vi "Update Custom Parameters.vi"(6 "Assert VI":path, 8 "error in (no error)":errorcluster, 10 "New Data Type":path) -> (0 "error out":errorcluster)   [LabVIEW 2018]
doc: "Updates the data types in the custom cluster data type, avoids having a whole set of extra type defs to maintain for the GTLT tests"
uses:
  <vilib>/Utility/traverseref.llb/TRef TravTarget.ctl
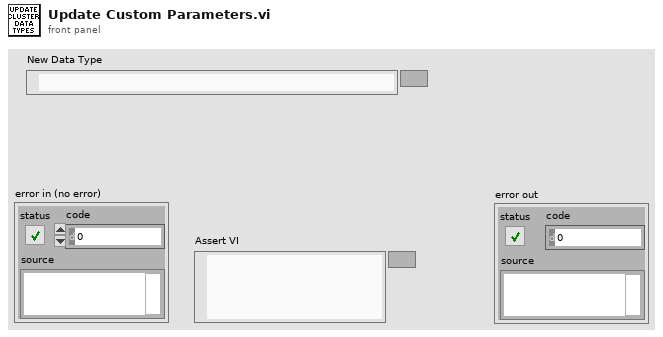
[diagram p1: front panel]
types:
  T1 = typedef "TRef TravTarget.ctl" = enum16{"FP", "BD", "Other"}
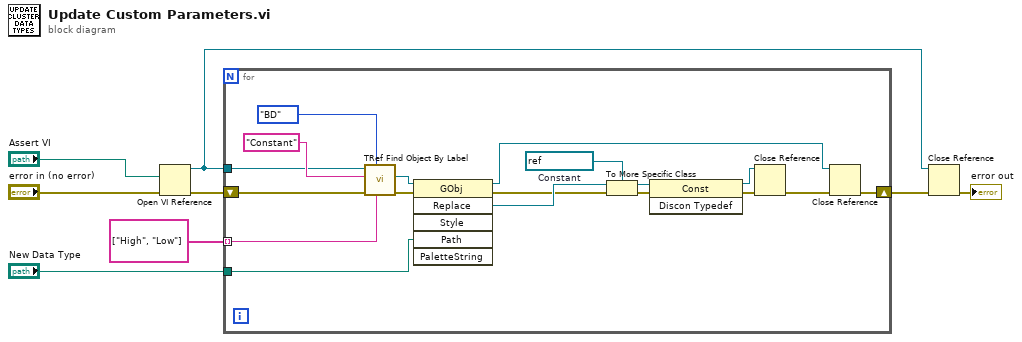
[diagram p0: block diagram]
diagram:
  n1 = Open VI Reference(vi path="Assert VI", error in (no error)="error in (no error)") -> (vi reference=w1:refnum<vi>, error out=w5:errorcluster)  [unwired: 4 in]
  n2 = for {
    tunnel: string[] ["High", "Low"] ("Label") -> [w26] mode=indexing
    tunnel: "New Data Type" -> [w21]
    tunnel: w1 -> [w9]
    shift-right: [w13] -> w3
    shift-left: w5 -> [w14]
    w19 = refnum<vi> refnum  # Constant
    n3 = call <vilib>:"TRef Find Object By Label.vi"("Label"=w26, "Traverse Target"=TRef_TravTarget."BD", "error in (no error)"=w14, "Class Name"="Constant", "VI Ref"=w9) -> ("error out"=w22:errorcluster, "Found Obj Ref"=w23:refnum<vi>)  [unwired: 3 in, 2 out]
    n4 = invoke class="GObj" method="Replace"(reference=w23, error in=w22, "Path"=w21) -> (reference out=w11:refnum<vi>, error out=w16:errorcluster, "Replace"=w20:refnum<vi>)  [unwired: 3 in, 3 out]
    n5 = To More Specific Class(target class=w19, reference=w20, error in=w16) -> (specific class reference=w18:refnum<vi>, error out=w17:errorcluster)
    n6 = invoke class="Const" method="Discon Typedef"(reference=w18, error in=w17) -> (reference out=w10:refnum<vi>, error out=w15:errorcluster)  [unwired: 1 in, 1 out]
    n7 = Close Reference(reference=w10, error in (no error)=w15) -> (error out=w12:errorcluster)
    n8 = Close Reference(reference=w11, error in (no error)=w12) -> (error out=w13:errorcluster)
  }
  n9 = Close Reference(reference=w1, error in (no error)=w3) -> (error out=→"error out":errorcluster)
